vi "Number_To_Fixed_Width_String.vi"(1 "Width":i32=6, 2 "Number":dbl) -> (0 "String":string)   [LabVIEW 2011]
doc: "This VI converts a given numerical value to a fixed-width string. For example, if the supplied value is 12.3 and the width is 6, the output will be 0012.3. If the supplied value is 1234.56, the output will be 1234.5."
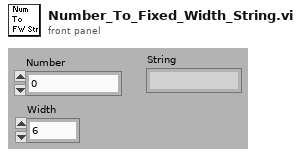
[diagram p1: front panel]
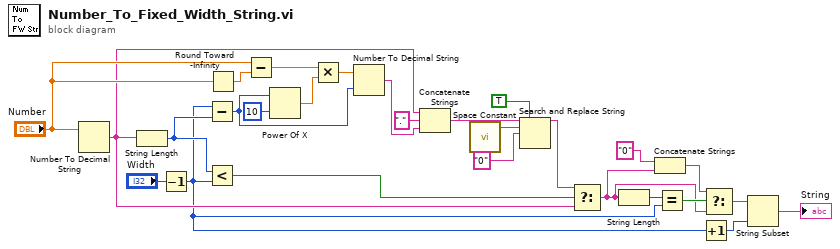
[diagram p0: block diagram]
diagram:
  n1 = Number To Decimal String(number="Number") -> (decimal integer string=w18:string)  [unwired: 1 out]
  n2 = String Length(string=w18) -> (length=w23:i32)
  n3 = Decrement(x="Width") -> (x-1=w3:i32)
  n4 = Subtract(x=w3, y=w23) -> (x-y=w16:i32)
  n5 = Less?(x=w23, y=w3) -> (x < y?=w20:bool)
  n6 = Round Toward -Infinity(1:"Number") -> (0:w26:dbl)
  n7 = Subtract(x="Number", y=w26) -> (x-y=w25:dbl)
  n8 = Power Of X(1:10 ("y"), 2:w16) -> (0:w24:dbl)
  n9 = Multiply(x=w25, y=w24) -> (x*y=w21:dbl)
  n10 = Number To Decimal String(number=w21, width (-)=w16) -> (decimal integer string=w17:string)
  n11 = Concatenate Strings(w18, "." ("string"), w17) -> (w12:string)
  n12 = call <vilib>:"Space Constant.vi"() -> ("String"=w15:string)
  n13 = Search and Replace String(replace all?=TRUE ("replace all? (F)"), input string=w12, search string=w15, replace string="0" ("replace string (\"\")")) -> (result string=w11:string)  [unwired: 1 in, 6 out]
  n14 = Select(t=w11, s=w20, f=w18) -> (s? t:f=w8:string)
  n15 = String Length(string=w8) -> (length=w10:i32)
  n16 = Concatenate Strings("0" ("string"), w8) -> (w7:string)
  n17 = Equal?(x=w10, y=w3) -> (x = y?=w9:bool)
  n18 = Increment(x=w3) -> (x+1=w2:i32)
  n19 = Select(t=w7, s=w9, f=w8) -> (s? t:f=w4:string)
  n20 = String Subset(string=w4, length (rest)=w2) -> (substring=→"String":string)  [unwired: 1 out]
